vi "Adresse Steuerung Kennung.vi"(8 "error in (no error)":errorcluster caption="Fehler (Eingang, kein Fehler)", 11 "Steuerung PNS Eingang":refnum<class "Steuerung PNS.lvclass">) -> (0 "error out":errorcluster caption="Fehler (Ausgang)", 2 "Adressen":T1, 3 "Steuerung PNS Ausgang":refnum<class "Steuerung PNS.lvclass">)   [LabVIEW 2020, in "Steuerung PNS.lvclass"]
uses:
  Steuerung PNS.lvclass
  Adresse.ctl
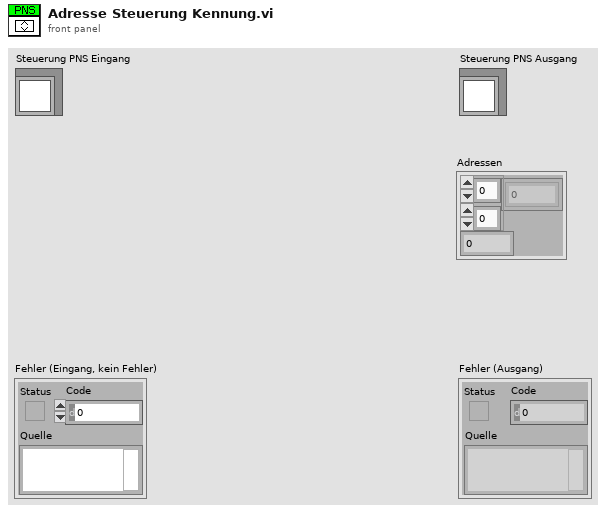
[diagram p1: front panel]
types:
  T1 = typedef "Steuerung PNS.lvclass/Adresse.ctl" = cluster{i32[][], i32}
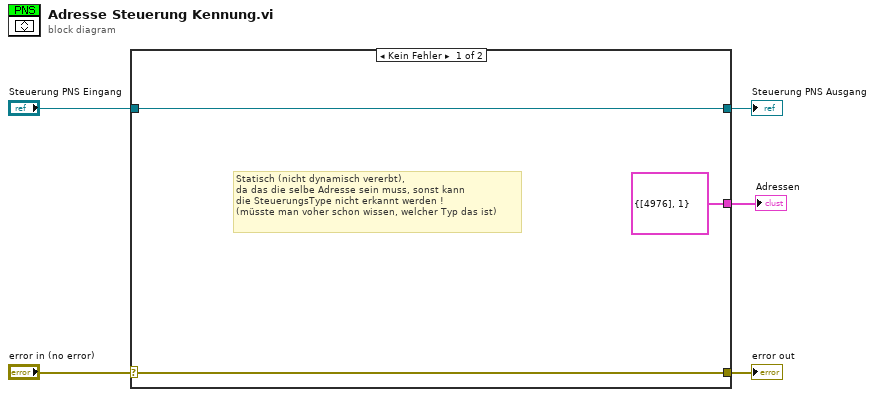
[diagram p0: block diagram]
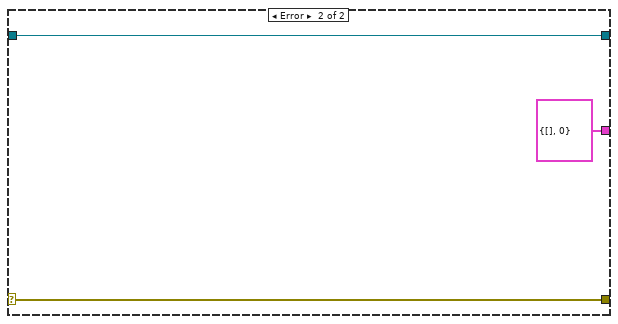
[diagram p2: hidden frame]
diagram:
  n1 = case shown="Kein Fehler" "error in (no error)" {
    selector: "error in (no error)" -> [w7 w11]
    tunnel: [w7 w11] -> w4
    tunnel: [w8 w10] -> w2
    tunnel: "Steuerung PNS Eingang" -> [w8 w10]
    tunnel: [T1 {[[4976]], 1} ("Adressen") T1 {[], 0} ("Adressen")] -> w1
    frame No Error {
      # "Statisch (nicht dynamisch vererbt),\nda das die selbe Adresse sein muss, sonst kann\ndie SteuerungsType nicht erkannt werden !\n(müsste man voher schon wissen, welcher Typ das ist)"
    }
    frame Error {
    }
  }
  "error out" <- w4
  "Steuerung PNS Ausgang" <- w2
  "Adressen" <- w1
